vi "Histogram-algo.vi"(5 "LSL":dbl, 7 "USL":dbl, 8 "error in":errorcluster, 10 "Data":dbl[](array[numeric])) -> (0 "error out":errorcluster, 3 "Histogram Graph":cluster{dbl[], dbl[]}[](graph))   [LabVIEW 2019, in "Zen Analytics.lvlib" / "Zen Analytics.lvclass"]
uses:
  Zen Analytics.lvclass
  <vilib>/Analysis/NI_AALPro.lvlib
  <vilib>/Analysis/NI_AALBase.lvlib
panel:
  out "Histogram Graph 3":T1(graph)
  out "Histogram Graph 2":cluster{"Histogram":i32[], "Axis":dbl[]}(graph)
  out "max value":i32
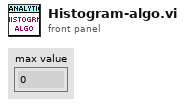
[diagram p1: front panel]
types:
  T1 = cluster{"X Values":dbl[], "Best Gaussian Fit":dbl[]}
  T2 = cluster{"Histogram: h(x)":i32[], "X Values":dbl[]}
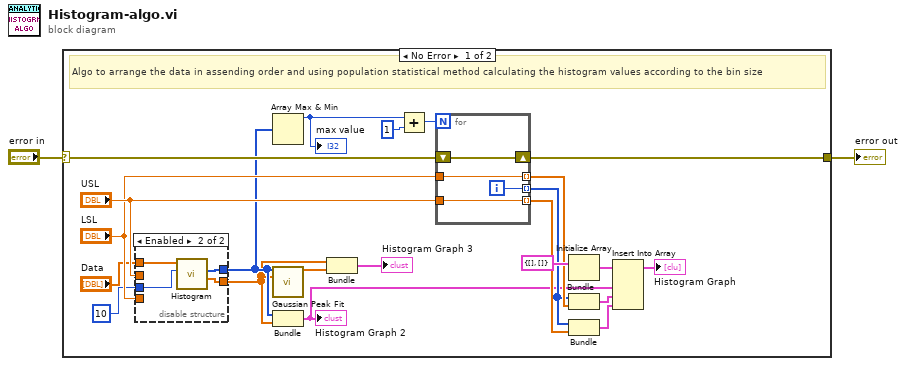
[diagram p0: block diagram]
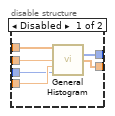
[diagram p2: hidden frame]
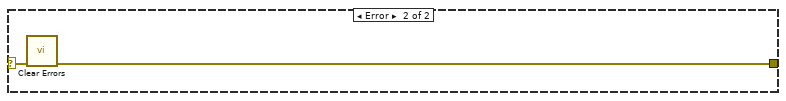
[diagram p3: hidden frame]
diagram:
  n1 = case shown="No Error" "error in" {
    selector: "error in" -> [w12 w40]
    tunnel: [w20 w39] -> w1
    frame No Error {
      # "Algo to arrange the data in assending order and using population statistical method calculating the histogram values according to the bin size"
      n2 = disable-structure shown="Enabled" {
        disable-tunnel: "Data" -> [w30 w34]
        disable-tunnel: "USL" -> [w29 _]
        disable-tunnel: "LSL" -> [w28 _]
        disable-tunnel: [w27 w32] -> w5
        disable-tunnel: [w26 w31] -> w4
        disable-tunnel: 10 ("# bins") -> [w25 w33]
        frame Disabled {
          n3 = call <vilib>:"General Histogram.vi"("X"=w30, "max"=w29, "min"=w28, "# bins"=w25) -> ("Histogram"=w27:i32[], "Axis"=w26:dbl[])  [unwired: 7 in, 3 out]
        }
        frame Enabled {
          n4 = call <vilib>:"Histogram.vi"("intervals"=w33, "X"=w34) -> ("X Values"=w31:dbl[], "Histogram: h(x)"=w32:i32[])  [unwired: 6 in, 2 out]
        }
      }
      n5 = Array Max & Min(array=w5) -> (max value=w15:i32)  [unwired: 3 out]
      "max value" <- w15
      n6 = call <vilib>:"Gaussian Peak Fit.vi"("Y"=w5, "X"=w4) -> ("Best Gaussian Fit"=w6:dbl[])  [unwired: 7 in, 6 out]
      n7 = Bundle("Histogram: h(x)"=w5, "X Values"=w4) -> (w9:T2)  [unwired: 1 in]
      "Histogram Graph 2" <- w9
      n8 = Bundle("X Values"=w4, "Best Gaussian Fit"=w6) -> (→"Histogram Graph 3":T1)  [unwired: 1 in]
      n9 = Add(x=w15, y=u32 1) -> (x+y=w14:u32)
      n10 = for {
        N: w14 -> [_]
        tunnel: "LSL" -> [w38]
        tunnel: [w38] -> w18 mode=indexing
        tunnel: "USL" -> [w37]
        tunnel: [w37] -> w17 mode=indexing
        tunnel: [w36] -> w16 mode=indexing
        shift-right: [w35] -> w20
        shift-left: w12 -> [w35]
        i -> [w36]
      }
      n11 = Initialize Array(cluster{dbl[], dbl[]} {[], []} ("output cluster")) -> (w24:cluster{dbl[], dbl[]}[])  [unwired: 1 in]
      n12 = Bundle(w16, w18) -> (w22:cluster{i32[], dbl[]})  [unwired: 1 in]
      n13 = Bundle(w16, w17) -> (w21:cluster{i32[], dbl[]})  [unwired: 1 in]
      n14 = Insert Into Array(array=w24, new element #1=w9, new element #2=w22, new element #3=w21) -> (→"Histogram Graph":cluster{dbl[], dbl[]}[])  [unwired: 1 in]
    }
    frame Error {
      n15 = call <vilib>:"Clear Errors.vi"("error in (no error)"=w40) -> ("error out"=w39:errorcluster)  [unwired: 5 in, 1 out]
    }
  }
  "error out" <- w1
